vi "AsignedUnasigned.vi"(5 "Days Open Phone Treshhold":dbl=0.01, 7 "AE Groups":T1(array[ring])=[enum."AE-Germany", enum."AE-Poland", enum."AE-Switzerland", enum."AE-Czech Republic", enum."AE-Hungary", enum."AE-Romania", enum."AE-Slovakia", enum."AE-Slovenia"], 8 "error in (no error)":errorcluster, 11 "All SR In":T2(array[cluster])) -> (0 "error out":errorcluster, 2 "Unassigned":T2(array[cluster]), 3 "Assigned Out":T2(array[cluster]))   [LabVIEW 2017, in "Client.lvlib" / "ParserSorter.lvlib"]
doc: "Check If Days Open > 0,1 and calculate Score based on Prio specific Base Values"
uses:
  ParserSorter.lvlib
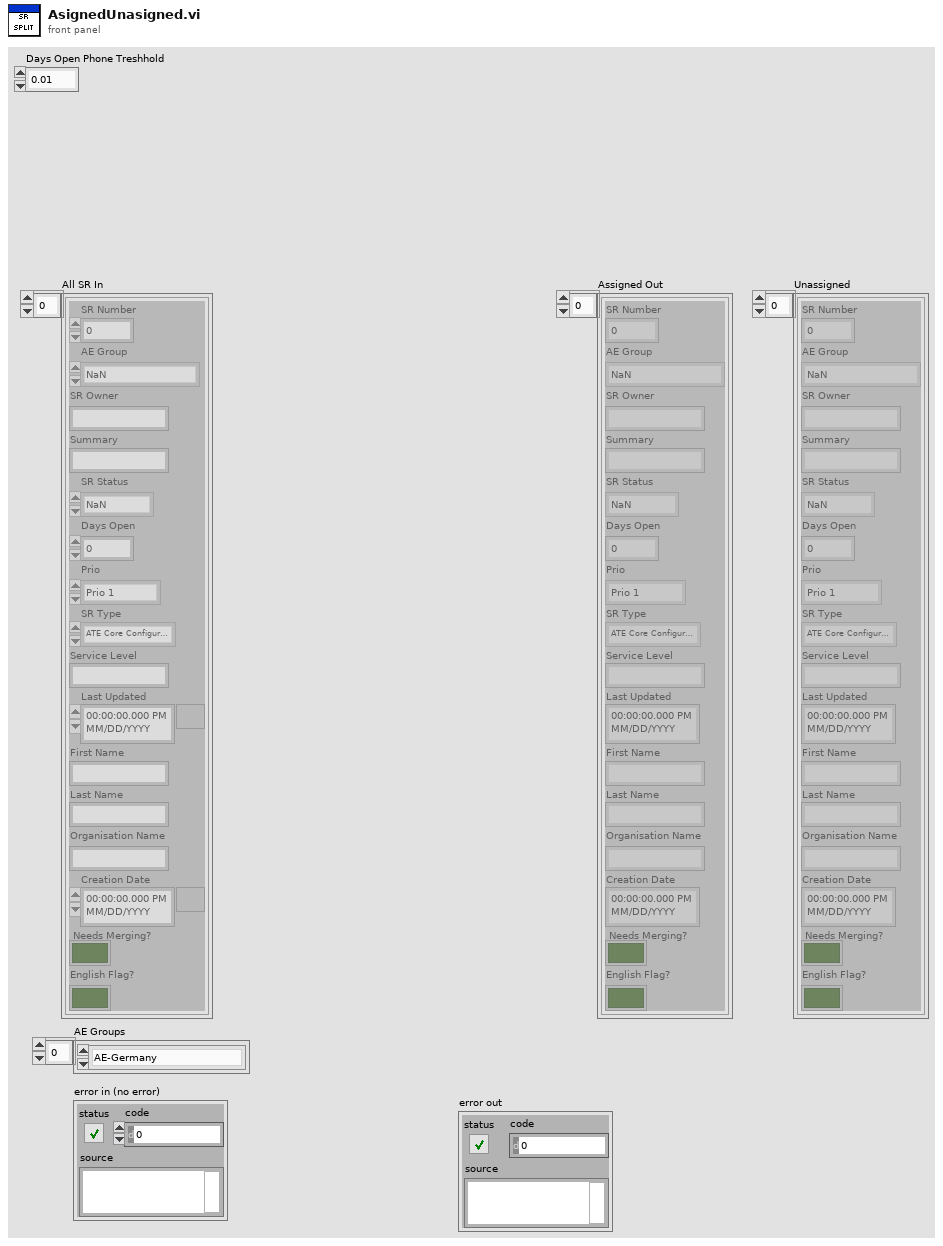
[diagram p1: front panel]
types:
  T1 = enum32{"NaN", "AE-Germany", "AE-Poland", "AE-Switzerland", "AE-Czech Republic", "AE-Hungary", "AE-Romania", "AE-Slovakia", "AE-Slovenia"}[]
  T2 = cluster{"SR Number":i64, "AE Group":enum32{"NaN", "AE-Germany", "AE-Poland", "AE-Switzerland", "AE-Czech Republic", "AE-Hungary", "AE-Romania", "AE-Slovakia", "AE-Slovenia"}, "SR Owner":string, "Summary":string, "SR Status":enum32{"NaN", "Caller Abandoned", "Created in Error", "Declined to Purchase Support", "Expired", "Forum Resolved AE", "Forum Resolved Customer", "IN WORK", "IN WORK Collab with AES", "IN WORK Collab with PSE", "IN WORK Collab with SE", "IN WORK Escalation", "IN WORK Customer Added Note", "Open", "Potentially Resolved", "POC Resolved", "Resolved", "RMA Waiting on Customer", "RMA Open", "RMA In Progress", "RMA Closed - DOA", "RMA Closed", "RMA Approved for Return", "Project Complete", "Presumed Resolved", "IN WORK Wait on Customer"}, "Days Open":dbl, "Prio":enum16{"Prio 1", "Prio 2", "Prio 3", "Prio 4"}, "SR Type":enum32{"NaN", "ATE Core Configurations (BYOATE)", "Activation", "BioBench", "CAN", "CM C Series", "Calibration", "Consulting Services", "CounterTimer", "DAQExpress", "DASYLab", "DIAdem", "DMM", "DSA HW", "Digital_IO", "FIRST (NIC Only)", "FieldBus", "FieldPoint", "Functional Savety", "GATI", "GPIB", "HMI and Industrial PCs", "HiQ", "HighSpeedDigital_IO", "IMAQ", "IOTech Vibration", "Industrial Communications", "InsightCM", "LV", "LV CD&Sim", "LV Comms", "LV Controls Add-Ons", "LV Embedded", "LV MathScript RT", "LV NXG", "LV NXT", "LVDSC", "LVFPGA", "LVPDA and LV Touch Panel", "LVRT", "LabWindows_CVI", "Lookout", "MATRIXx", "MStudioDotNet", "MStudioVisualBasic", "MStudioVisualC", "Measure (Legacy)", "Motion", "MultifunctionDAQ", "Multimedia Test HW/SW", "Multisim (EWB)", "NI Update Service", "OPC Servers", "Optical (OSI)", "PXI Controllers, Chassis, MXI", "PXI Timing and Sync", "Power Supplies and SMUs", "Powertrain Controls", "RAID", "RF", "RF Software", "RIO", "SC Express", "SCC", "SCXI", "SPEEDY-33 (Hyperception)", "STS", "ScopeDigitizers", "Serial", "Signal Sources", "SignalCondOther", "SignalExpress", "Software Defined Intruments", "Sound and Vibration SW", "Switch Executive", "Switches", "TestStand", "USRP", "Ultiboard (EWB)", "VBench", "VI Logger", "VXI_MXI", "VeriStand", "VisionSW", "VolumeLicenseMgr", "WSN", "Web UI Builder", "myRIO"}, "Service Level":string, "Last Updated":timestamp, "First Name":string, "Last Name":string, "Organisation Name":string, "Creation Date":timestamp, "Needs Merging?":bool, "English Flag?":bool}[]
  T3 = cluster{"SR Number":i64, "AE Group":enum32{"NaN", "AE-Germany", "AE-Poland", "AE-Switzerland", "AE-Czech Republic", "AE-Hungary", "AE-Romania", "AE-Slovakia", "AE-Slovenia"}, "SR Owner":string, "Summary":string, "SR Status":enum32{"NaN", "Caller Abandoned", "Created in Error", "Declined to Purchase Support", "Expired", "Forum Resolved AE", "Forum Resolved Customer", "IN WORK", "IN WORK Collab with AES", "IN WORK Collab with PSE", "IN WORK Collab with SE", "IN WORK Escalation", "IN WORK Customer Added Note", "Open", "Potentially Resolved", "POC Resolved", "Resolved", "RMA Waiting on Customer", "RMA Open", "RMA In Progress", "RMA Closed - DOA", "RMA Closed", "RMA Approved for Return", "Project Complete", "Presumed Resolved", "IN WORK Wait on Customer"}, "Days Open":dbl, "Prio":enum16{"Prio 1", "Prio 2", "Prio 3", "Prio 4"}, "SR Type":enum32{"NaN", "ATE Core Configurations (BYOATE)", "Activation", "BioBench", "CAN", "CM C Series", "Calibration", "Consulting Services", "CounterTimer", "DAQExpress", "DASYLab", "DIAdem", "DMM", "DSA HW", "Digital_IO", "FIRST (NIC Only)", "FieldBus", "FieldPoint", "Functional Savety", "GATI", "GPIB", "HMI and Industrial PCs", "HiQ", "HighSpeedDigital_IO", "IMAQ", "IOTech Vibration", "Industrial Communications", "InsightCM", "LV", "LV CD&Sim", "LV Comms", "LV Controls Add-Ons", "LV Embedded", "LV MathScript RT", "LV NXG", "LV NXT", "LVDSC", "LVFPGA", "LVPDA and LV Touch Panel", "LVRT", "LabWindows_CVI", "Lookout", "MATRIXx", "MStudioDotNet", "MStudioVisualBasic", "MStudioVisualC", "Measure (Legacy)", "Motion", "MultifunctionDAQ", "Multimedia Test HW/SW", "Multisim (EWB)", "NI Update Service", "OPC Servers", "Optical (OSI)", "PXI Controllers, Chassis, MXI", "PXI Timing and Sync", "Power Supplies and SMUs", "Powertrain Controls", "RAID", "RF", "RF Software", "RIO", "SC Express", "SCC", "SCXI", "SPEEDY-33 (Hyperception)", "STS", "ScopeDigitizers", "Serial", "Signal Sources", "SignalCondOther", "SignalExpress", "Software Defined Intruments", "Sound and Vibration SW", "Switch Executive", "Switches", "TestStand", "USRP", "Ultiboard (EWB)", "VBench", "VI Logger", "VXI_MXI", "VeriStand", "VisionSW", "VolumeLicenseMgr", "WSN", "Web UI Builder", "myRIO"}, "Service Level":string, "Last Updated":timestamp, "First Name":string, "Last Name":string, "Organisation Name":string, "Creation Date":timestamp, "Needs Merging?":bool, "English Flag?":bool}
  T4 = enum32{"NaN", "AE-Germany", "AE-Poland", "AE-Switzerland", "AE-Czech Republic", "AE-Hungary", "AE-Romania", "AE-Slovakia", "AE-Slovenia"}
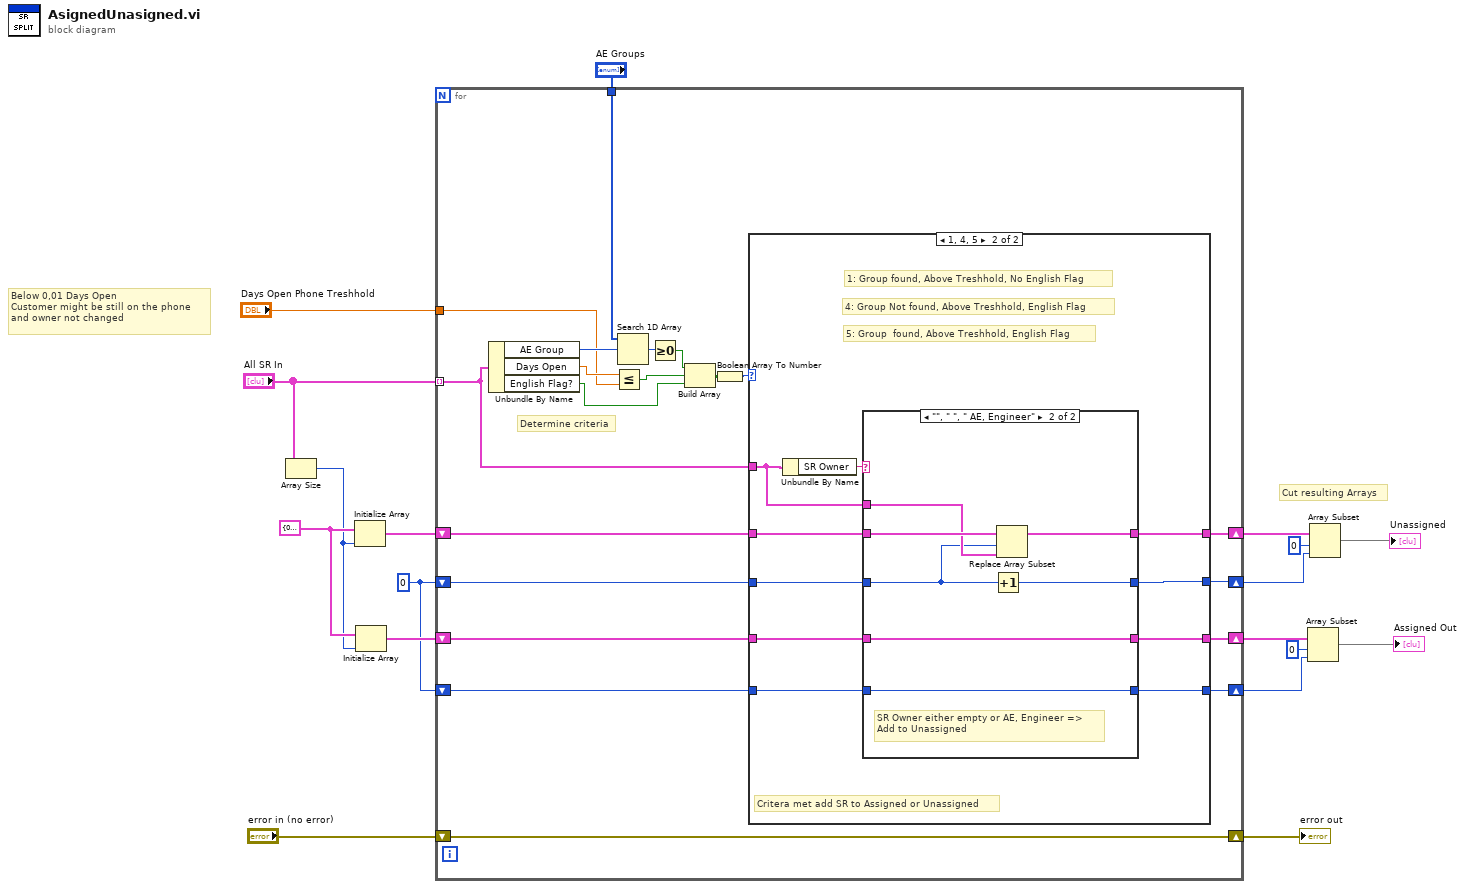
[diagram p0: block diagram]
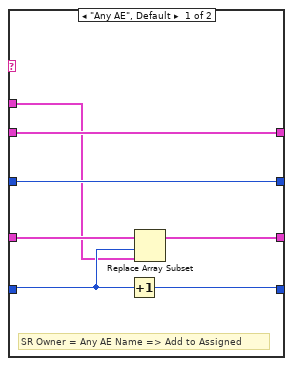
[diagram p3: hidden frame]
diagram:
  w11 = 0 ("size(s)")
  w15 = T3 {"SR Number"=0, "AE Group"=enum."NaN", "SR Owner"="", "Summary"="", "SR Status"=enum."NaN", "Days Open"=0.0, "Prio"=enum."Prio 1", "SR Type"=enum."ATE Core Configurations (BYOATE)", "Service Level"="", "Last Updated"=timestamp(0 s since 1904-01-01), "First Name"="", "Last Name"="", "Organisation Name"="", "Creation Date"=timestamp(0 s since 1904-01-01), "Needs Merging?"=FALSE, "English Flag?"=FALSE} ("SR Number")
  # "Below 0,01 Days Open\nCustomer might be still on the phone\nand owner not changed"
  # "Cut resulting Arrays"
  n1 = Array Size(array="All SR In") -> (size(s)=w14:i32)
  n2 = Initialize Array(w15, w14) -> (w12:T2)
  n3 = Initialize Array(w15, w14) -> (w13:T2)
  n4 = for {
    shift-right: [w38] -> w17
    shift-left: "error in (no error)" -> [w38]
    tunnel: "All SR In" -> [w35] mode=indexing
    shift-right: [w33] -> w6
    shift-left: w12 -> [w37]
    shift-right: [w32] -> w10
    shift-left: w13 -> [w31]
    shift-right: [w34] -> w3
    shift-left: w11 -> [w36]
    shift-right: [w30] -> w2
    shift-left: w11 -> [w29]
    tunnel: "Days Open Phone Treshhold" -> [w23]
    tunnel: "AE Groups" -> [w21]
    # "Determine criteria"
    n5 = Unbundle By Name(w35) -> ("AE Group"=w28:T4, "Days Open"=w24:dbl, "English Flag?"=w27:bool)
    n6 = Less Or Equal?(x=w24, y=w23) -> (x <= y?=w22:bool)
    n7 = Search 1D Array(1D array=w21, element=w28) -> (index of element=w20:i32)  [unwired: 1 in]
    n8 = Greater Or Equal To 0?(x=w20) -> (x >= 0?=w19:bool)
    n9 = Build Array(w19, w22, w27) -> (w25:bool[])
    n10 = Boolean Array To Number(Boolean array=w25) -> (number=w26:u32)
    n11 = case shown="1, 4, 5" w26 {
      tunnel: w37 -> [w42 w51]
      tunnel: w36 -> [w41 w49]
      tunnel: w35 -> [_ w43]
      tunnel: [w41 w45] -> w34
      tunnel: [w42 w44] -> w33
      tunnel: [w40 w46] -> w32
      tunnel: w31 -> [w40 w50]
      tunnel: [w39 w47] -> w30
      tunnel: w29 -> [w39 w48]
      frame 0, 2, 3, 6, 7, Default {
        # "6: Group Not found, Below Treshhold, No English Flag"
        # "7: Group  found, Below Treshhold,  English Flag"
        # "3: Group  found, Below Treshhold, No English Flag"
        # "2: Group Not found, Below Treshhold, No English Flag"
        # "Criteria not met, dont add to SR list"
      }
      frame 1, 4, 5 {
        # "5: Group  found, Above Treshhold, English Flag"
        # "4: Group Not found, Above Treshhold, English Flag"
        # "1: Group found, Above Treshhold, No English Flag"
        # "Critera met add SR to Assigned or Unassigned"
        n12 = Unbundle By Name(w43) -> ("SR Owner"=w52:string)
        n13 = case shown="\"\", \" \", \" AE, Engineer\"" w52 {
          tunnel: w51 -> [w55 w66]
          tunnel: w49 -> [w54 w63]
          tunnel: w50 -> [w59 w60]
          tunnel: w48 -> [w56 w61]
          tunnel: [w55 w65] -> w44
          tunnel: w43 -> [w53 w64]
          tunnel: [w54 w62] -> w45
          tunnel: [w57 w61] -> w47
          tunnel: [w58 w60] -> w46
          frame "Any AE", Default {
            # "SR Owner = Any AE Name => Add to Assigned"
            n14 = Increment(x=w56) -> (x+1=w57:i32)
            n15 = Replace Array Subset(array=w59, new element=w53, index=w56) -> (w58:T2)
          }
          frame "", " ", " AE, Engineer" {
            # "SR Owner either empty or AE, Engineer => \nAdd to Unassigned"
            n16 = Increment(x=w63) -> (x+1=w62:i32)
            n17 = Replace Array Subset(array=w66, new element=w64, index=w63) -> (w65:T2)
          }
        }
      }
    }
  }
  "error out" <- w17
  n18 = Array Subset(array=w10, index=0, length=w2) -> (→"Assigned Out":T2)
  n19 = Array Subset(array=w6, index=0, length=w3) -> (→"Unassigned":T2)
